vi "init.vi"(8 "error in (no error)":errorcluster, 10 "Resource":string, 11 "ScopeKeysight in":refnum<class "ScopeKeysight.lvclass">) -> (0 "error out":errorcluster, 3 "ScopeKeysight out":refnum<class "ScopeKeysight.lvclass">)   [LabVIEW 2023, in "ScopeKeysight.lvclass"]
doc: "Initialize the instrument by a given resource string or alias name"
uses:
  ScopeKeysight.lvclass
  ScopeKeysight.lvclass/ScopeKeysight.ctl
  Scope.lvclass
  Driver/Keysight-DSQx3014T.lvlib
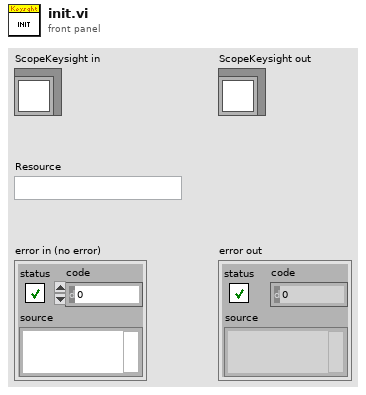
[diagram p1: front panel]
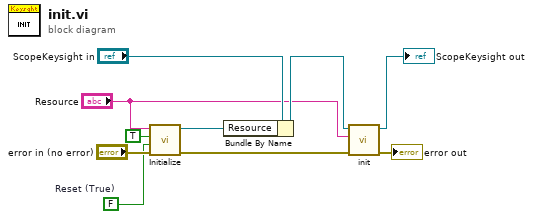
[diagram p0: block diagram]
diagram:
  w1 = FALSE  # Reset (True)
  n1 = call "Initialize.vi"("error in (no error)"="error in (no error)", "Reset (True)"=w1, "ID Query (True)"=TRUE, "VISA resource name"="Resource") -> ("error out"=w5:errorcluster, "VISA resource name out"=w6:refnum<visa-resource-name>)  [unwired: 6 in]
  n2 = Bundle By Name(cluster="ScopeKeysight in", "Resource"=w6) -> (w7:refnum<class "ScopeKeysight.lvclass">)
  n3 = call-parent "init.vi"("error in (no error)"=w5, "Resource"="Resource", "Instrument in"=w7) -> ("error out"=→"error out":errorcluster, "Instrument out"=→"ScopeKeysight out":refnum<class "ScopeKeysight.lvclass">)  [unwired: 7 in]
